vi "Post - Any Class.vi"(7 "PV name":string, 8 "error in (no error)":errorcluster, 10 "value in":refnum<class "Base Interface.lvclass">, 11 "Server in":refnum<class "Server.lvclass">) -> (0 "error out":errorcluster, 2 "value out":refnum<class "Base Interface.lvclass">, 3 "Server out":refnum<class "Server.lvclass">)   [LabVIEW 2020, in "PV Access.lvlib" / "PVA Server.lvlib" / "Server.lvclass"]
uses:
  Server.lvclass
  Server.lvclass/Server.ctl
  Source/Source.lvclass
  PV Data/Base Interface/Base Interface.lvclass
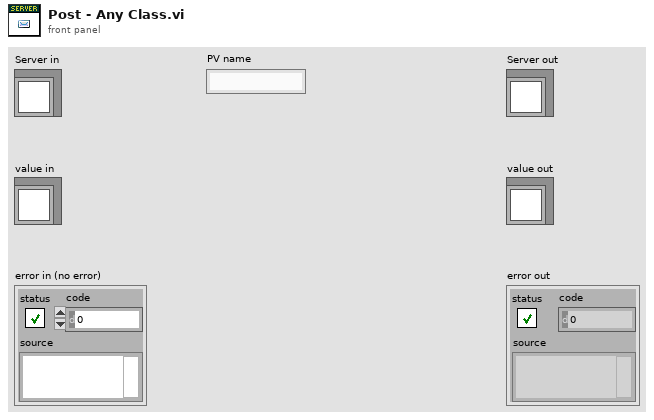
[diagram p1: front panel]
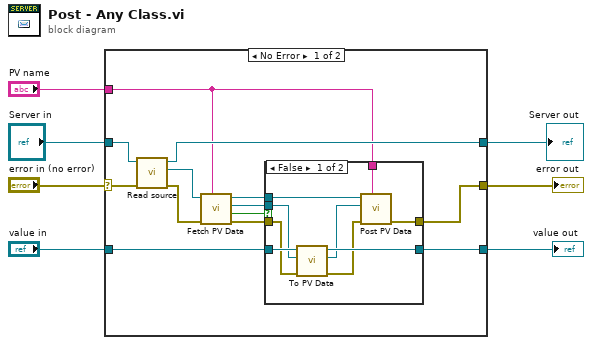
[diagram p0: block diagram]
diagram:
  n1 = case shown="No Error" "error in (no error)" {
    selector: "error in (no error)" -> [w13 w34]
    tunnel: [w14 w34] -> w4
    tunnel: [w19 w33] -> w3
    tunnel: "Server in" -> [w20 w33]
    tunnel: "PV name" -> [w15 _]
    tunnel: "value in" -> [w17 w32]
    tunnel: [w18 w32] -> w1
    frame No Error {
      n2 = call "Read source.vi"("error in (no error)"=w13, "Server in"=w20) -> ("error out"=w12:errorcluster, "Source"=w16:refnum<class "Source.lvclass">, "Server out"=w19:refnum<class "Server.lvclass">)  [unwired: 7 in]
      n3 = call "Fetch PV Data.vi"("PV name"=w15, "error in"=w12, "Source in"=w16) -> ("error out"=w10:errorcluster, "PV not found?"=w8:bool, "PV Data out"=w9:refnum<class "PV Data.lvclass">, "Source out"=w11:refnum<class "Source.lvclass">)  [unwired: 5 in]
      n4 = case shown="False" w8 {
        tunnel: [w29 w30] -> w18
        tunnel: w17 -> [w28 w30]
        tunnel: w15 -> [w27 _]
        tunnel: [w26 w31] -> w14
        tunnel: w11 -> [w25 _]
        tunnel: w10 -> [w23 w31]
        tunnel: w9 -> [w22 _]
        frame False {
          n5 = call-dynamic "To PV Data.vi"("error in"=w23, "PV data in"=w22, "Base Interface in"=w28) -> ("error out"=w24:errorcluster, "PV data out"=w21:refnum<class "PV Data.lvclass">, "Base Interface out"=w29:refnum<class "Base Interface.lvclass">)  [unwired: 6 in]
          n6 = call "Post PV Data.vi"("PV name"=w27, "error in"=w24, "PV Data in"=w21, "Source in"=w25) -> ("error out"=w26:errorcluster)  [unwired: 6 in, 1 out]
        }
        frame True {
        }
      }
    }
    frame Error {
    }
  }
  "error out" <- w4
  "Server out" <- w3
  "value out" <- w1
